vi "TravZSurveySubVI.vi"() -> ()   [LabVIEW 2022 SP3]
uses:
  Gen Trav/Trav_mode.ctl
  Globals/Trav_pos_global.vi
  <vilib>/Utility/file.llb/Write To Spreadsheet File (string).vi
panel:
  in  "Note":string
  in  "logfile path (dialog if empty)":path
  out "AngleXYZ":dbl[](array[numeric]) caption="Angle                    X                    Y                   Z" format="%.1f"
  out "Z sensor (mm)":dbl format="%.1g"
  out "String":string
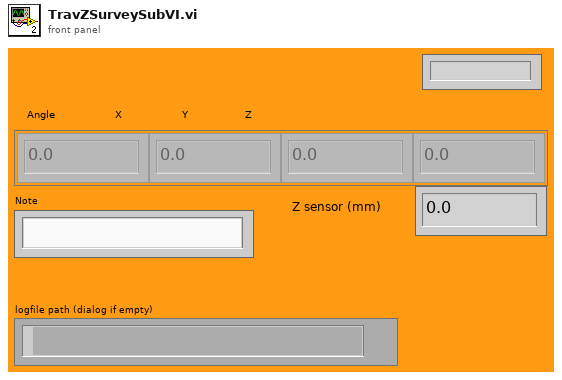
[diagram p1: front panel]
types:
  T1 = typedef "Trav_mode.ctl" = enum16{"Move traverse", "Read traverse position", "Teach Position"}
  T2 = typedef "AxisConfigCluster.ctl" = cluster{"Channel Properties":T3, "Static Drive Configuration":T4}
  T3 = typedef "DriveProperties.ctl" = cluster{"Channel Name":string, "Vel. Default":sgl, "Acc. Default":sgl, "Vel. Max":sgl, "Vel. Min":sgl, "Acc. Max":sgl, "Acc. Min":sgl, "Pulses/unit":sgl, "Address":u8, "Pulse Offset":i32, "Pos Tolerance":sgl, "Pulses/rev":sgl, "Backlash/Eng units":sgl, "Current Pos":sgl, "Ch Status":enum16{"Active", "Offline", "Simulate"}, "Port Name":string, "Axis Transform mode":string, "Metadata Ch Name":string, "Type":string}
  T4 = typedef "DriveStaticConfig.ctl" = cluster{"Correction Gain % (CG)":u16, "Dead Band (DB)":i32, "Dead Band Window (DW)":i32, "Encoder Resolution (ER)":i32, "Step Mode  (FSB)":u16, "Position Maintenance (FSC)":u16, "Stop on Stall (FSD)":u16, "Activate OP1 on stall (FSE)":u16, "Stop on Trigger 3 (FSF)":u16, "OP2 in Deadband (FSG)":u16, "Stall Detect (FSH)":u16, "Limit Disable (LD)":u16, "Motor Resolution (MR)":enum16{"200", "400", "1000", "2000", "4000", "5000", "10000", "12800", "18000", "20000", "21600", "25000", "25400", "25600", "36000", "50000", "278528", "425984", "507904", "614400", "655360", "819200", "1024000"}, "Limit Switch Sense (OSA)":u16, "Home Position (OSB)":u16, "Home Switch Sense (OSC)":u16, "Encoder Z for Home (OSD)":u16, "Reference edge of Home (OSH)":u16, "RS232 Echo Control (SSA)":u16, "Buffer at Limit (SSG)":u16, "Buffer at Stop (SSH)":u16, "Indexer Mode  (FSA)":u16, "Type":string, "ConfigString":string, "De Power Motor":enum16{"TRUE", "FALSE"}}
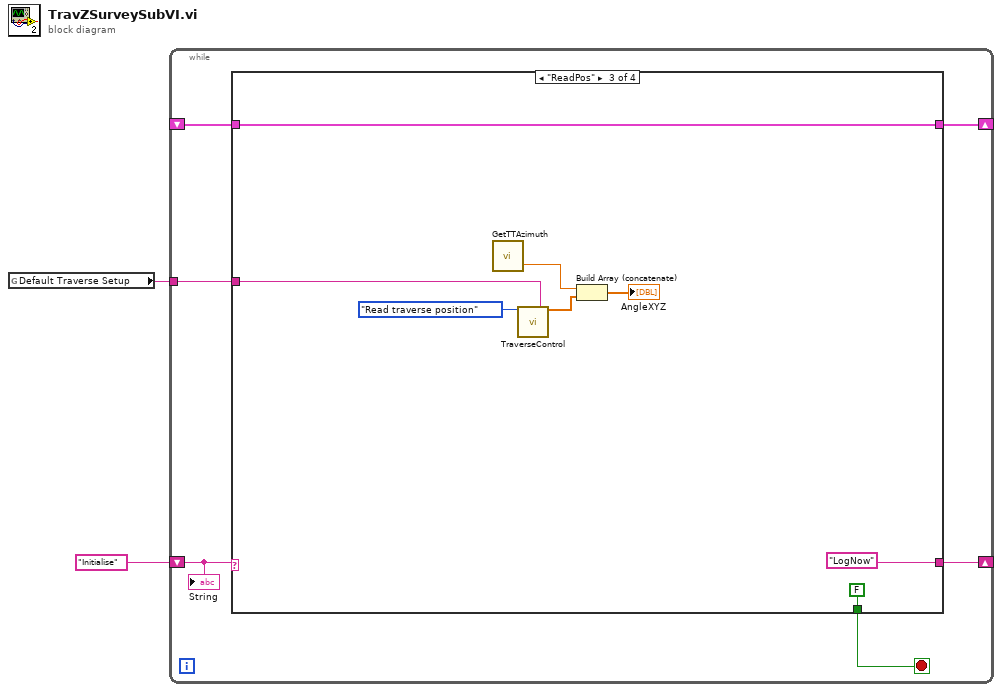
[diagram p0: block diagram]
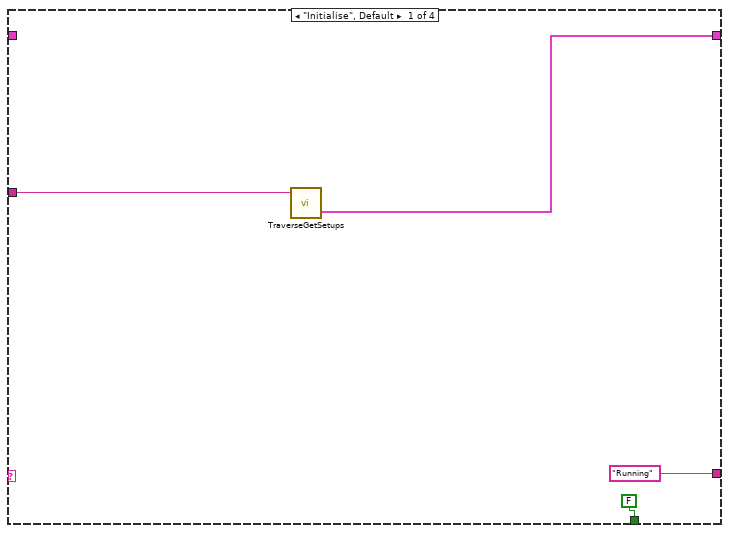
[diagram p2: hidden frame]
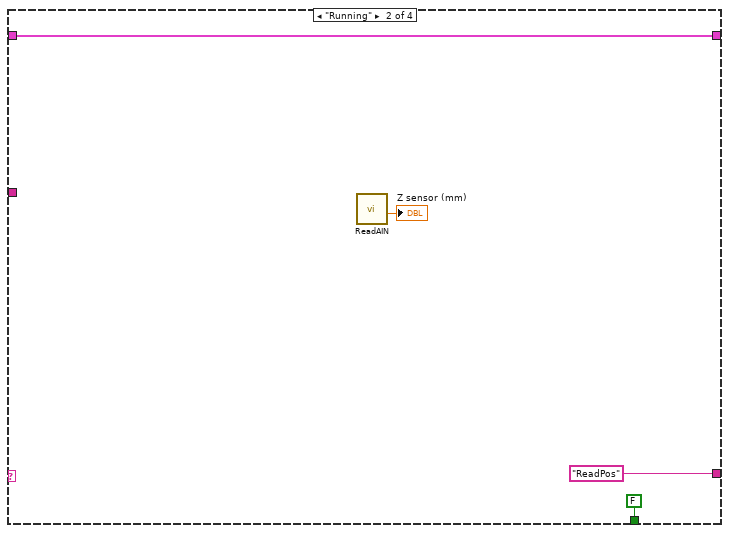
[diagram p3: hidden frame]
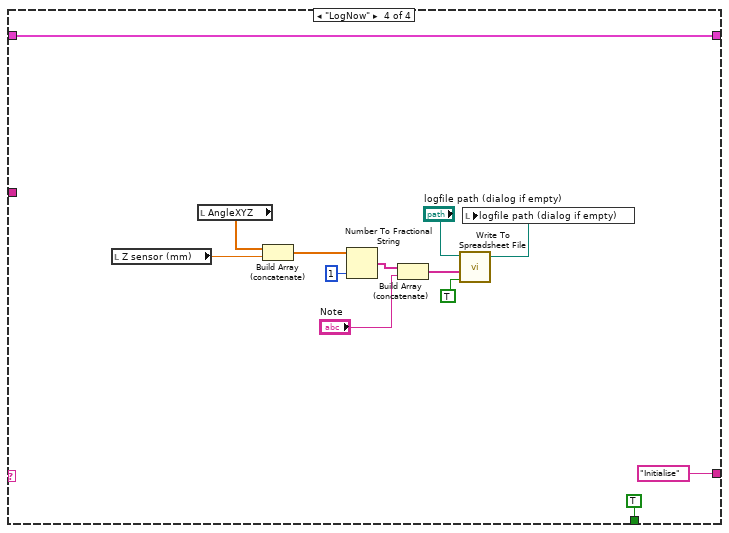
[diagram p4: hidden frame]
diagram:
  n1 = global read "Trav_pos_global.vi" "Default Traverse Setup"() -> (w1:string)
  n2 = while {
    shift-right: [w6] -> _
    shift-left: "Initialise" -> [w8]
    tunnel: w1 -> [w7]
    shift-right: [w5] -> _
    shift-left: _ -> [w4]
    stop <- w3 stop-if-true
    n3 = case shown="\"ReadPos\"" w8 {
      tunnel: w7 -> [w12 _ w18 _]
      tunnel: ["Running" "ReadPos" "LogNow" "Initialise"] -> w6
      tunnel: [w11 w16 w24 w37] -> w5
      tunnel: w4 -> [_ w16 w24 w37]
      tunnel: [FALSE FALSE FALSE TRUE] -> w3
      frame "Initialise", Default {
        n4 = call "TraverseGetSetups.vi"("Traverse Name"=w12) -> ("Matched Configurations"=w11:T2[])  [unwired: 2 in, 1 out]
      }
      frame "Running" {
        n5 = call "ReadAIN.vi"() -> ("mm"=→"Z sensor (mm)":dbl)  [unwired: 10 in, 1 out]
      }
      frame "ReadPos" {
        n6 = call "GetTTAzimuth.vi"() -> ("TurntableAngle"=w19:dbl)  [unwired: 2 in, 1 out]
        n7 = call "TraverseControl.vi"("Mode"=Trav_mode."Read traverse position", "Traverse Name"=w18) -> ("Position Output XYZ"=w20:sgl[])  [unwired: 15 in, 2 out]
        n8 = Build Array (concatenate)(w19, w20) -> (→"AngleXYZ":dbl[])
      }
      frame "LogNow" {
        n9 = local read "Z sensor (mm)"() -> (w27:dbl)
        n10 = local read "AngleXYZ"() -> (w28:dbl[])
        n11 = Build Array (concatenate)(w28, w27) -> (w31:dbl[])
        n12 = Number To Fractional String(number=w31, precision (6)=i16 1) -> (F-format string=w35:string[])  [unwired: 2 out]
        n13 = Build Array (concatenate)(w35, "Note") -> (w34:string[])
        n14 = call-poly <vilib>:"Write To Spreadsheet File.vi"("append to file? (new file:F)"=TRUE, "1D data"=w34, "file path (dialog if empty)"="logfile path (dialog if empty)") -> ("new file path (Not A Path if cancelled)"=w29:path)  [unwired: 3 in, 2 out]
        n15 = local write "logfile path (dialog if empty)"(w29) -> ()
      }
    }
    "String" <- w8
  }
